vi "PhotonCamera_GetDriverMode.vi"(9 "BaseNTName":string="/photonvision", 11 "CameraName":string) -> (0 "error out":errorcluster, 3 "DriverMode":bool)   [LabVIEW 2019, in "PhotonVisionLib.lvlib"]
doc: "Returns whether the camera is in driver mode.\n\nInputs:\n - CameraName -- The nickname of the camera (found in the PhotonVision UI).\n - BaseNTName - string - Base Nework Table name. (Optional. Default: /photonvision )\n \nOutputs:\n - DriverMode -- Boolean indicating whether the camera is in driver mode.\n - Error Out -- Contains error information if a Network table ot other error occured."
uses:
  PhotonVisionLib.lvlib
  <vilib>/Rock Robotics/Network Tables/NT Read Boolean.vi
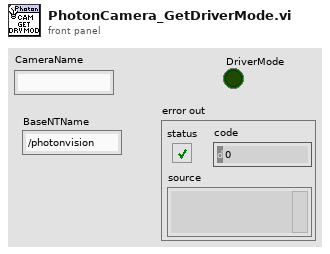
[diagram p1: front panel]
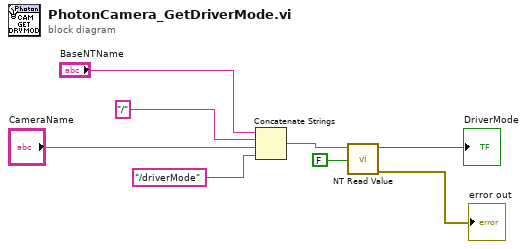
[diagram p0: block diagram]
diagram:
  n1 = Concatenate Strings("BaseNTName", "/", "CameraName", "/driverMode") -> (w5:string)
  n2 = call-poly <vilib>:"NT Read Value.vi"("default value"=FALSE ("Default Value"), "name"=w5) -> ("error out"=→"error out":errorcluster, "value"=→"DriverMode":bool)  [unwired: 7 in, 1 out]
